vi "DC-RMS per Channel.vi"(4 "Array Length":i32, 6 "Measurement Control":T1(array[cluster]) {"exp. time constant" format="%0.2p"}, 7 "reset":bool, 8 "error in (no error)":errorcluster, 9 "Averaging Time":dbl[](array[numeric]) format="%0.2p", 10 "Enable":bool[](array[boolean]), 11 "signals in":waveform(dbl)[](array[waveform])) -> (0 "error out":errorcluster, 2 "data ready":bool, 3 "DC value waveforms":waveform(dbl)[](array[waveform]))   [LabVIEW 2017]
uses:
  <vilib>/measure/NI_MAPro.lvlib
  <vilib>/measure/NI_MABase.lvlib
panel:
  in  "averaging type":enum16{"Linear", "Exponential"}(ring)
  out "measurements info":T2(array[cluster]) {"uncertainty" format="%0.2p"}
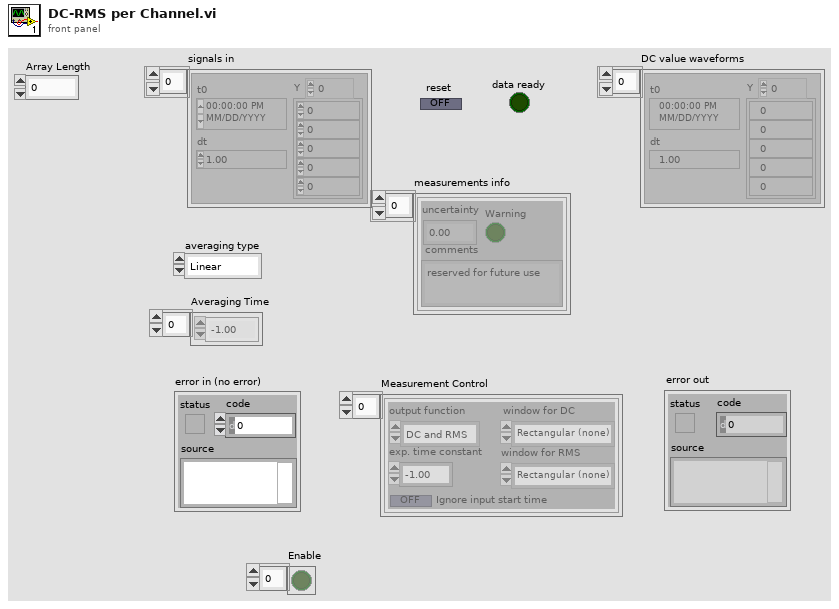
[diagram p1: front panel]
types:
  T1 = cluster{"window for DC":enum16{"Rectangular (none)", "Hanning", "Low side lobe"}, "output function":enum16{"DC only", "RMS only", "DC and RMS"}, "window for RMS":enum16{"Rectangular (none)", "Hanning", "Low side lobe"}, "exp. time constant":dbl, "Ignore input start time":bool}[]
  T2 = cluster{"uncertainty":dbl, "Warning":bool, "comments":string}[]
  T3 = cluster{"DC history":dbl, "RMS history":dbl, "exp TC (samples)":dbl, "buffer size":i32, "t0 history":timestamp, "dt history":dbl, "timestamp":timestamp, "buffer":dbl[]}
  T4 = cluster{"uncertainty":dbl, "Warning":bool, "comments":string}
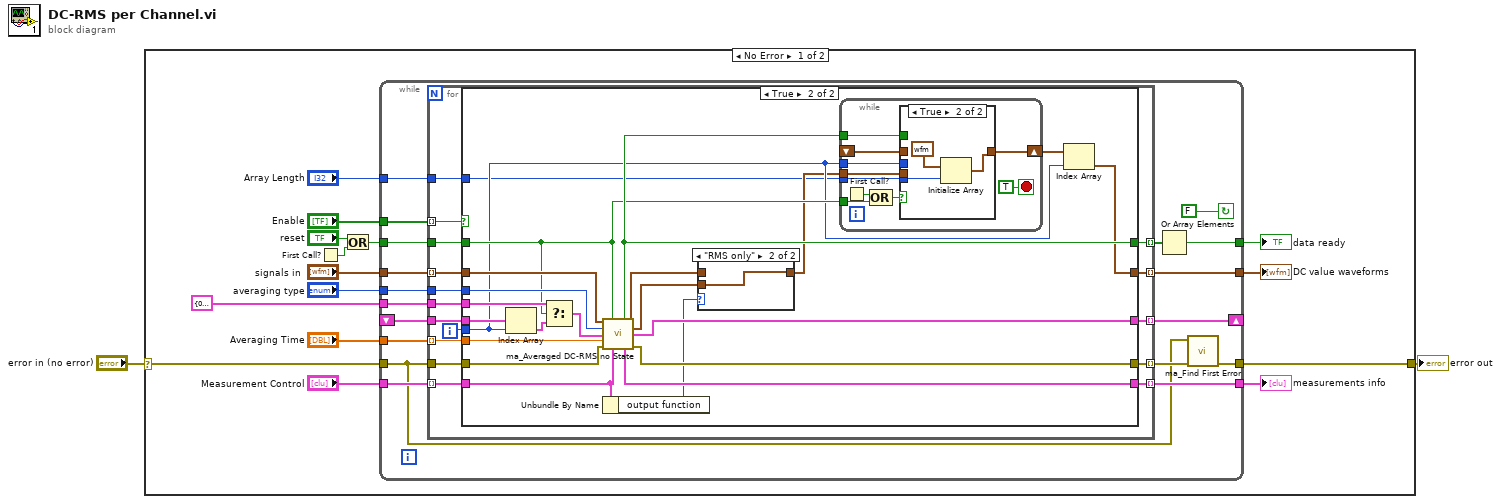
[diagram p0: block diagram]
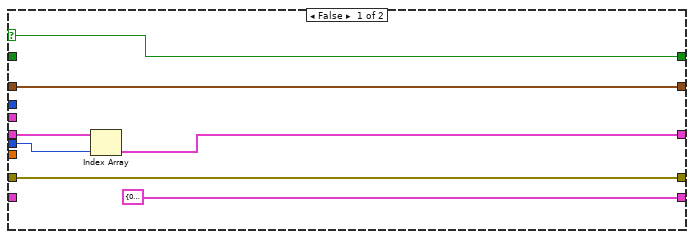
[diagram p2: hidden frame]
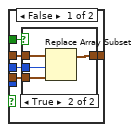
[diagram p3: hidden frame]
diagram:
  n1 = case shown="No Error" "error in (no error)" {
    selector: "error in (no error)" -> [w8 w106]
    tunnel: [w9 w106] -> w2
    frame No Error {
      n2 = First Call?() -> (First Call?: T/F=w15:bool)
      n3 = Or(x="reset", y=w15) -> (x .or. y?=w14:bool)
      n4 = while {
        tunnel: [w23] -> w10
        tunnel: "Measurement Control" -> [w28]
        tunnel: T3 {"DC history"=0.0, "RMS history"=0.0, "exp TC (samples)"=0.0, "buffer size"=0, "t0 history"=timestamp(0 s since 1904-01-01), "dt history"=0.0, "timestamp"=timestamp(0 s since 1904-01-01), "buffer"=[]} ("state info") -> [w24]
        shift-left: _ -> [w25]
        shift-right: [w31] -> _
        tunnel: w8 -> [w20]
        tunnel: "averaging type" -> [w35]
        tunnel: [w29] -> w12
        tunnel: "signals in" -> [w27]
        tunnel: "Averaging Time" -> [w33]
        tunnel: [w34] -> w17
        tunnel: w14 -> [w26]
        tunnel: [w21] -> w9
        tunnel: "Enable" -> [w19]
        tunnel: "Array Length" -> [w18]
        stop <- FALSE continue-if-true
        n5 = for {
          tunnel: w35 -> [w50]
          tunnel: [w44] -> w34 mode=indexing
          tunnel: w33 -> [w48] mode=indexing
          tunnel: w27 -> [w49] mode=indexing
          tunnel: [w45] -> w32 mode=indexing
          tunnel: w25 -> [w41]
          tunnel: [w51] -> w31 mode=indexing
          tunnel: w26 -> [w39]
          tunnel: w28 -> [w43] mode=indexing
          tunnel: w24 -> [w40]
          tunnel: [w38] -> w23 mode=indexing
          tunnel: w20 -> [w47]
          tunnel: [w46] -> w22 mode=indexing
          tunnel: w19 -> [w37] mode=indexing
          tunnel: w18 -> [w36]
          i -> [w42]
          n6 = case shown="True" w37 {
            selector: w37 -> [w52 _]
            tunnel: [w54 w80] -> w51
            tunnel: w50 -> [_ w79]
            tunnel: w49 -> [w58 w78]
            tunnel: w48 -> [_ w77]
            tunnel: w47 -> [w57 w76]
            tunnel: [w57 w75] -> w46
            tunnel: [w52 w65] -> w45
            tunnel: [w58 w61] -> w44
            tunnel: w43 -> [_ w69]
            tunnel: w42 -> [w55 w62]
            tunnel: w41 -> [w56 w72]
            tunnel: w40 -> [_ w71]
            tunnel: w39 -> [_ w64]
            tunnel: [T4 {"uncertainty"=0.0, "Warning"=FALSE, "comments"=""} ("measurement info cluster") w70] -> w38
            tunnel: w36 -> [_ w59]
            frame False {
              n7 = Index Array(array=w56, index=w55) -> (element=w54:T3)
            }
            frame True {
              n8 = Index Array(array=w72, index=w62) -> (element=w74:T3)
              n9 = Select(t=w71, s=w64, f=w74) -> (s? t:f=w73:T3)
              n10 = call <vilib>:"ma_Averaged DC-RMS no State.vi"("signal in"=w78, "reset"=w64, "averaging type"=w79, "state info"=w73, "averaging time"=w77, "error in"=w76, "averaging control"=w69) -> ("data ready"=w65:bool, "DC value waveform"=w67:waveform(dbl), "RMS value waveform"=w66:waveform(dbl), "state info"=w80:T3, "measurement info cluster"=w70:T4, "error out"=w75:errorcluster)  [unwired: 3 in]
              n11 = Unbundle By Name(w69) -> ("output function"=w68:enum16{"DC only", "RMS only", "DC and RMS"})
              n12 = case shown="\"RMS only\"" w68 {
                tunnel: [w104 w105] -> w60
                tunnel: w67 -> [w104 _]
                tunnel: w66 -> [_ w105]
                frame "DC only", Default {
                }
                frame "RMS only" {
                }
              }
              n13 = while {
                shift-right: [w89] -> w63
                shift-left: _ -> [w88]
                tunnel: w65 -> [w87]
                tunnel: w59 -> [w85]
                tunnel: w62 -> [w84]
                tunnel: w60 -> [w83]
                tunnel: w64 -> [w81]
                stop <- TRUE stop-if-true
                n14 = First Call?() -> (First Call?: T/F=w86:bool)
                n15 = Compound Arithmetic op=OR(w86, w81) -> (w82:bool)
                n16 = case shown="True" w82 {
                  tunnel: [w95 w101] -> w89
                  tunnel: w88 -> [w94 _]
                  tunnel: w87 -> [w93 _]
                  tunnel: w85 -> [_ w102]
                  tunnel: w84 -> [w92 _]
                  tunnel: w83 -> [w91 _]
                  frame False {
                    n17 = case shown="True" w93 {
                      tunnel: [w96 w99] -> w95
                      tunnel: w94 -> [w96 w100]
                      tunnel: w92 -> [_ w98]
                      tunnel: w91 -> [_ w97]
                      frame False {
                      }
                      frame True {
                        n18 = Replace Array Subset(array=w100, new element=w97, index=w98) -> (w99:waveform(dbl)[])
                      }
                    }
                  }
                  frame True {
                    n19 = Initialize Array(waveform(dbl) {"t0"=timestamp(0 s since 1904-01-01), "dt"=1.0, "Y"=[]} ("element"), w102) -> (w101:waveform(dbl)[])
                  }
                }
              }
              n20 = Index Array(array=w63, index=w62) -> (element=w61:waveform(dbl))
            }
          }
        }
        n21 = Or Array Elements(Boolean array=w32) -> (logical OR=w29:bool)
        n22 = call <vilib>:"ma_Find First Error.vi"("error array in"=w22, "error in 1 (no error)"=w20) -> ("error out"=w21:errorcluster)  [unwired: 5 in]
      }
      "data ready" <- w12
      "DC value waveforms" <- w17
      "measurements info" <- w10
    }
    frame Error {
    }
  }
  "error out" <- w2
